vi "desmontaCabecalho.vi"(7 "cabeçalho":u8 format="%.0x") -> (6 "addr":u8 format="%.0x", 10 "opcode":u8 format="%.0x")   [LabVIEW 2018]
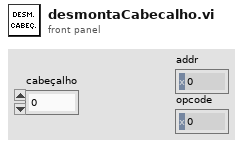
[diagram p1: front panel]
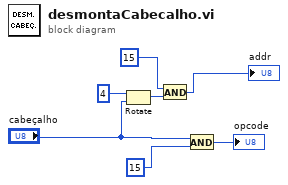
[diagram p0: block diagram]
diagram:
  n1 = Rotate(1:"cabeçalho", 2:i16 4 ("y")) -> (0:w3:u8)
  n2 = And(x=u8 15, y=w3) -> (x .and. y?=→"addr":u8)
  n3 = And(x="cabeçalho", y=u8 15) -> (x .and. y?=→"opcode":u8)
